vi "Report Digital Command.vi"(6 "Value":bool, 8 "error in (no error)":errorcluster, 9 "Name":string, 10 "VolatusAPI in":refnum<class "VolatusAPI.lvclass">, 11 "GUI Element in":refnum<class "GUI Element.lvclass">) -> (0 "error out":errorcluster, 3 "GUI Element out":refnum<class "GUI Element.lvclass">)   [LabVIEW 2020, in "VolatusGUI.lvlib" / "GUI Element.lvclass"]
uses:
  GUI Element.lvclass
  GUI Element.lvclass/GUI Element.ctl
  Volatus/VolatusAPI/VolatusAPI.lvclass
  lv-vecto/Vecto/Vecto.lvlib
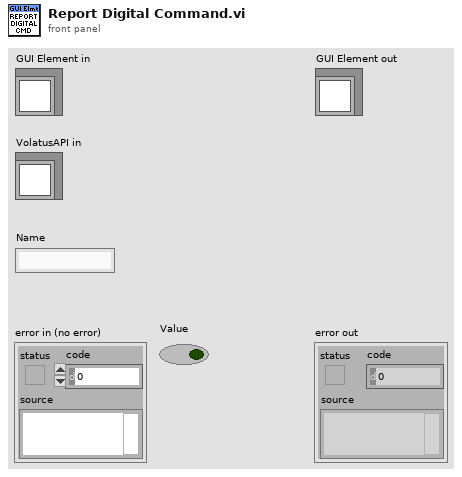
[diagram p1: front panel]
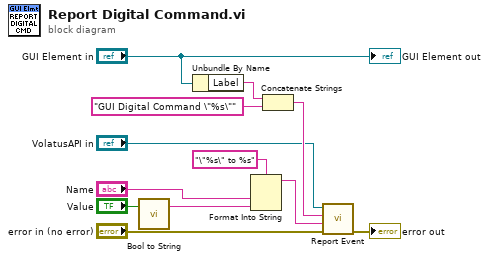
[diagram p0: block diagram]
diagram:
  n1 = call "Bool to String.vi"("Bool"="Value") -> ("String"=w5:string)  [unwired: 2 in]
  n2 = Unbundle By Name("GUI Element in") -> ("Label"=w8:string)
  n3 = Format Into String(format string="\"%s\" to %s", "Name", w5) -> (resulting string=w3:string)  [unwired: 2 in, 1 out]
  n4 = Concatenate Strings(w8, "GUI Digital Command \"%s\"" ("string")) -> (w7:string)
  n5 = call "Report Event.vi"("error in (no error)"="error in (no error)", "Message"=w3, "Context"=w7, "VolatusAPI in"="VolatusAPI in") -> ("error out"=→"error out":errorcluster)  [unwired: 6 in, 1 out]
  "GUI Element out" <- "GUI Element in"
